vi "FGV cRIO-Daten.vi"(0 "cRIO DI - DO":u32[](array[numeric]), 1 "Analog Input":T4, 2 "TC Eingänge":T1, 3 "Stickstoff Befüllung":dbl[](array[numeric]), 4 "Störungen":u64[](array[numeric]), 5 "CPU Status":sgl[](array[numeric]), 7 "PID Stellwerte":i16[](array[numeric]), 11 "Aktion":enum16{"lesen", "schreiben"}(ring)) -> (6 "DI":T3, 10 "DO 0-31":T5, 12 "DO 32-63":T2, 13 "PID Stellwerte":i16[](array[numeric]), 14 "Betriebsstunden":sgl[](array[numeric]), 15 "Analog Input":T4, 16 "TC Eingänge":T1, 17 "Stickstoff Befüllung":dbl[](array[numeric]), 18 "Störungen":u64[](array[numeric]), 19 "CPU Status":sgl[](array[numeric]))   [LabVIEW 2020, in "Kommunikation mit cRIO.lvlib"]
uses:
  Kommunikation mit cRIO.lvlib
  Verwaltung/Analog Eingaenge.ctl
  Verwaltung/Digital Ausgaenge 0-31.ctl
  Verwaltung/Digital Eingaenge 0-15.ctl
  Verwaltung/Digital Ausgaenge 32-63.ctl
  Verwaltung/TC Eingaenge.ctl
  Verwaltung/Verwaltung - cRIO.lvlib
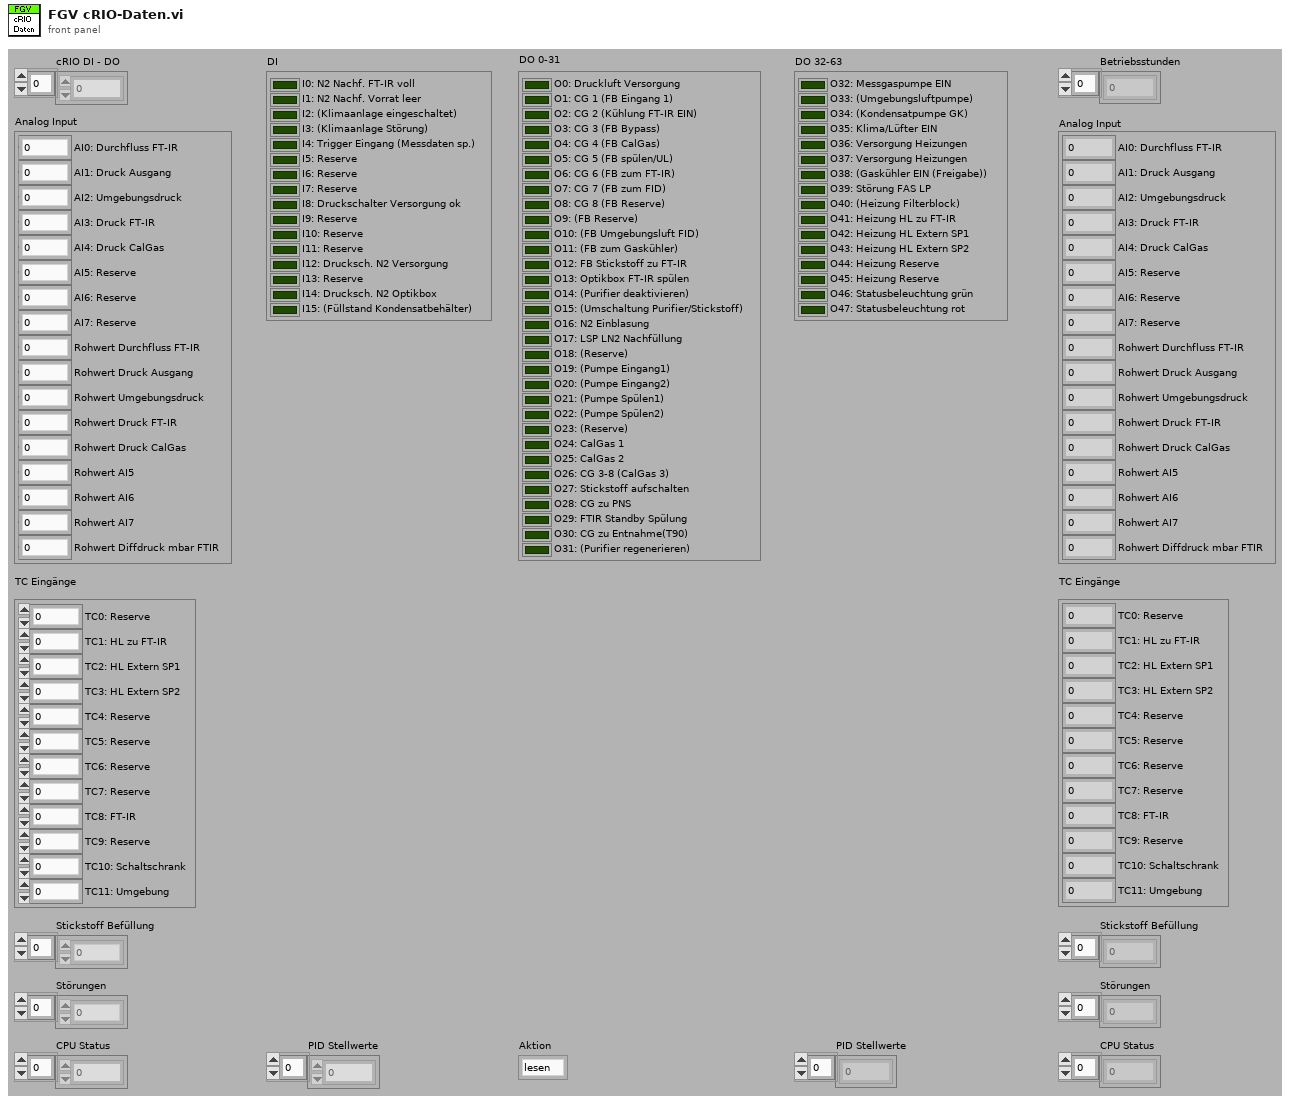
[diagram p1: front panel]
types:
  T1 = typedef "Verwaltung - cRIO.lvlib/TC Eingaenge.ctl" = cluster{"TC0: Reserve":sgl, "TC1: HL zu FT-IR":sgl, "TC2: HL Extern SP1":sgl, "TC3: HL Extern SP2":sgl, "TC4: Reserve":sgl, "TC5: Reserve":sgl, "TC6: Reserve":sgl, "TC7: Reserve":sgl, "TC8: FT-IR":sgl, "TC9: Reserve":sgl, "TC10: Schaltschrank":sgl, "TC11: Umgebung":sgl}
  T2 = typedef "Verwaltung - cRIO.lvlib/Digital Ausgaenge 32-63.ctl" = cluster{"O32: Messgaspumpe EIN":bool, "O33: (Umgebungsluftpumpe)":bool, "O34: (Kondensatpumpe GK)":bool, "O35: Klima/Lüfter EIN":bool, "O36: Versorgung Heizungen":bool, "O37: Versorgung Heizungen":bool, "O38: (Gaskühler EIN (Freigabe))":bool, "O39: Störung FAS LP":bool, "O40: (Heizung Filterblock)":bool, "O41: Heizung HL zu FT-IR":bool, "O42: Heizung HL Extern SP1":bool, "O43: Heizung HL Extern SP2":bool, "O44: Heizung Reserve":bool, "O45: Heizung Reserve":bool, "O46: Statusbeleuchtung grün":bool, "O47: Statusbeleuchtung rot":bool}
  T3 = typedef "Verwaltung - cRIO.lvlib/Digital Eingaenge 0-15.ctl" = cluster{"I0: N2 Nachf. FT-IR voll":bool, "I1: N2 Nachf. Vorrat leer":bool, "I2: (Klimaanlage eingeschaltet)":bool, "I3: (Klimaanlage Störung)":bool, "I4: Trigger Eingang (Messdaten sp.)":bool, "I5: Reserve":bool, "I6: Reserve":bool, "I7: Reserve":bool, "I8: Druckschalter Versorgung ok":bool, "I9: Reserve":bool, "I10: Reserve":bool, "I11: Reserve":bool, "I12: Drucksch. N2 Versorgung":bool, "I13: Reserve":bool, "I14: Drucksch. N2 Optikbox":bool, "I15: (Füllstand Kondensatbehälter)":bool}
  T4 = typedef "Verwaltung - cRIO.lvlib/Analog Eingaenge.ctl" = cluster{"AI0: Durchfluss FT-IR":sgl, "AI1: Druck Ausgang":sgl, "AI2: Umgebungsdruck":sgl, "AI3: Druck FT-IR":sgl, "AI4: Druck CalGas":sgl, "AI5: Reserve":sgl, "AI6: Reserve":sgl, "AI7: Reserve":sgl, "Rohwert Durchfluss FT-IR":sgl, "Rohwert Druck Ausgang":sgl, "Rohwert Umgebungsdruck":sgl, "Rohwert Druck FT-IR":sgl, "Rohwert Druck CalGas":sgl, "Rohwert AI5":sgl, "Rohwert AI6":sgl, "Rohwert AI7":sgl, "Rohwert Diffdruck mbar FTIR":sgl}
  T5 = typedef "Verwaltung - cRIO.lvlib/Digital Ausgaenge 0-31.ctl" = cluster{"O0: Druckluft Versorgung":bool, "O1: CG 1 (FB Eingang 1)":bool, "O2: CG 2 (Kühlung FT-IR EIN)":bool, "O3: CG 3 (FB Bypass)":bool, "O4: CG 4 (FB CalGas)":bool, "O5: CG 5 (FB spülen/UL)":bool, "O6: CG 6 (FB zum FT-IR)":bool, "O7: CG 7 (FB zum FID)":bool, "O8: CG 8 (FB Reserve)":bool, "O9: (FB Reserve)":bool, "O10: (FB Umgebungsluft FID)":bool, "O11: (FB zum Gaskühler)":bool, "O12: FB Stickstoff zu FT-IR":bool, "O13: Optikbox FT-IR spülen":bool, "O14: (Purifier deaktivieren)":bool, "O15: (Umschaltung Purifier/Stickstoff)":bool, "O16: N2 Einblasung":bool, "O17: LSP LN2 Nachfüllung":bool, "O18: (Reserve)":bool, "O19: (Pumpe Eingang1)":bool, "O20: (Pumpe Eingang2)":bool, "O21: (Pumpe Spülen1)":bool, "O22: (Pumpe Spülen2)":bool, "O23: (Reserve)":bool, "O24: CalGas 1":bool, "O25: CalGas 2":bool, "O26: CG 3-8 (CalGas 3)":bool, "O27: Stickstoff aufschalten":bool, "O28: CG zu PNS":bool, "O29: FTIR Standby Spülung":bool, "O30: CG zu Entnahme(T90)":bool, "O31: (Purifier regenerieren)":bool}
  T6 = cluster{"Boolean array[0]":bool, "Boolean array[1]":bool, "Boolean array[2]":bool, "Boolean array[3]":bool, "Boolean array[4]":bool, "Boolean array[5]":bool, "Boolean array[6]":bool, "Boolean array[7]":bool, "Boolean array[8]":bool, "Boolean array[9]":bool, "Boolean array[10]":bool, "Boolean array[11]":bool, "Boolean array[12]":bool, "Boolean array[13]":bool, "Boolean array[14]":bool, "Boolean array[15]":bool}
  T7 = cluster{"Boolean array[0]":bool, "Boolean array[1]":bool, "Boolean array[2]":bool, "Boolean array[3]":bool, "Boolean array[4]":bool, "Boolean array[5]":bool, "Boolean array[6]":bool, "Boolean array[7]":bool, "Boolean array[8]":bool, "Boolean array[9]":bool, "Boolean array[10]":bool, "Boolean array[11]":bool, "Boolean array[12]":bool, "Boolean array[13]":bool, "Boolean array[14]":bool, "Boolean array[15]":bool, "Boolean array[16]":bool, "Boolean array[17]":bool, "Boolean array[18]":bool, "Boolean array[19]":bool, "Boolean array[20]":bool, "Boolean array[21]":bool, "Boolean array[22]":bool, "Boolean array[23]":bool, "Boolean array[24]":bool, "Boolean array[25]":bool, "Boolean array[26]":bool, "Boolean array[27]":bool, "Boolean array[28]":bool, "Boolean array[29]":bool, "Boolean array[30]":bool, "Boolean array[31]":bool}
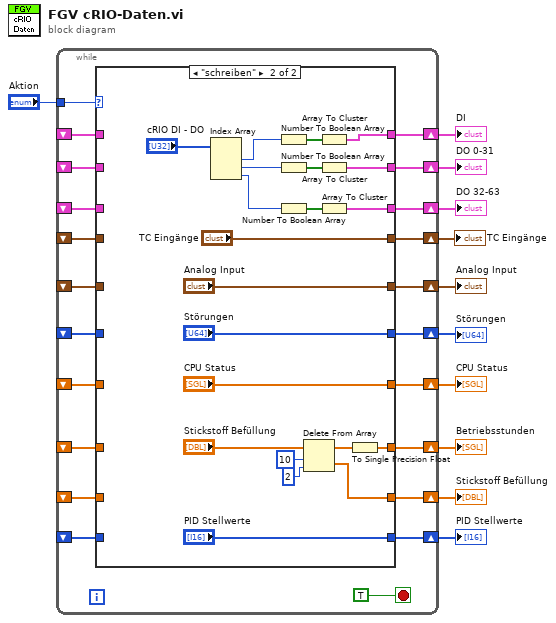
[diagram p0: block diagram]
diagram:
  n1 = while {
    tunnel: "Aktion" -> [w33]
    shift-right: [w31] -> w10
    shift-left: _ -> [w29]
    shift-right: [w30] -> w9
    shift-left: _ -> [w28]
    shift-right: [w26] -> w7
    shift-left: _ -> [w24]
    shift-right: [w27] -> w8
    shift-left: _ -> [w25]
    shift-right: [w23] -> w6
    shift-left: _ -> [w22]
    shift-right: [w21] -> w5
    shift-left: _ -> [w19]
    shift-right: [w20] -> w4
    shift-left: _ -> [w18]
    shift-right: [w17] -> w3
    shift-left: _ -> [w16]
    shift-right: [w15] -> w2
    shift-left: _ -> [w14]
    shift-right: [w13] -> w1
    shift-left: _ -> [w12]
    stop <- TRUE stop-if-true
    n2 = case shown="\"schreiben\"" w33 {
      tunnel: [w43 "Analog Input"] -> w31
      tunnel: [w42 "Störungen"] -> w30
      tunnel: w29 -> [w43 _]
      tunnel: w28 -> [w42 _]
      tunnel: [w41 w59] -> w27
      tunnel: [w40 w56] -> w26
      tunnel: w25 -> [w41 _]
      tunnel: w24 -> [w40 _]
      tunnel: [w39 "CPU Status"] -> w23
      tunnel: w22 -> [w39 _]
      tunnel: [w38 w52] -> w21
      tunnel: [w37 w46] -> w20
      tunnel: w19 -> [w38 _]
      tunnel: w18 -> [w37 _]
      tunnel: [w36 "PID Stellwerte"] -> w17
      tunnel: w16 -> [w36 _]
      tunnel: [w35 w45] -> w15
      tunnel: w14 -> [w35 _]
      tunnel: [w34 "TC Eingänge"] -> w13
      tunnel: w12 -> [w34 _]
      frame "lesen", Default {
      }
      frame "schreiben" {
        n3 = Index Array(array="cRIO DI - DO") -> (element #1=w61:u32, element #2=w57:u32, element #3=w53:u32)  [unwired: 3 in]
        n4 = Number To Boolean Array(number=w61) -> (Boolean array=w60:bool[])
        n5 = Number To Boolean Array(number=w57) -> (Boolean array=w58:bool[])
        n6 = Number To Boolean Array(number=w53) -> (Boolean array=w54:bool[])
        n7 = Delete From Array(array="Stickstoff Befüllung", length=10 ("Länge"), index=2 ("Index")) -> (deleted portion=w46:dbl[], array with subset deleted=w50:dbl[])
        n8 = Array To Cluster(array=w60) -> (cluster=w59:T6)
        n9 = Array To Cluster(array=w58) -> (cluster=w56:T7)
        n10 = Array To Cluster(array=w54) -> (cluster=w52:T6)
        n11 = To Single Precision Float(number=w50) -> (single precision float=w45:sgl[])
      }
    }
  }
  "Analog Input" <- w10
  "DO 0-31" <- w7
  "Störungen" <- w9
  "DI" <- w8
  "CPU Status" <- w6
  "DO 32-63" <- w5
  "Stickstoff Befüllung" <- w4
  "PID Stellwerte" <- w3
  "Betriebsstunden" <- w2
  "TC Eingänge" <- w1
